vi "4_5.vi"() -> ()   [LabVIEW 2012]
panel:
  in  "stop":bool
  in  "OK Button":bool
  out "-":dbl[](array[numeric])
  out "+":dbl[](array[numeric])
  in  "Array":dbl[](array[numeric])
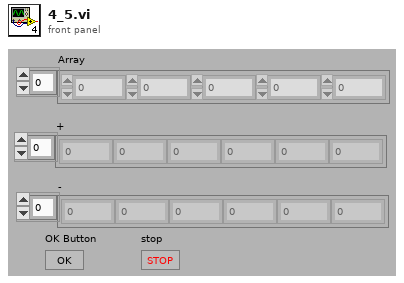
[diagram p1: front panel]
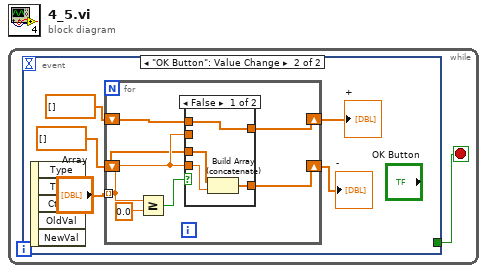
[diagram p0: block diagram]
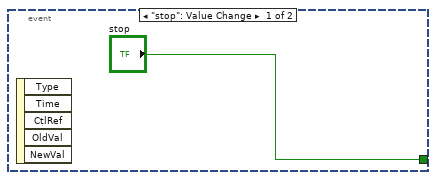
[diagram p2: hidden frame]
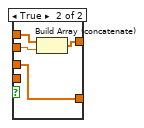
[diagram p3: hidden frame]
diagram:
  n1 = while {
    stop <- w1 stop-if-true
    n2 = event shown="[1] \"OK Button\": Value Change" {
      selector: _ -> [_ _]
      dyn-events: _ -> [_ _]
      timeout: _ -> [_ _]
      tunnel: ["stop" _] -> w1
      event "stop": Value Change {
        n3 = event-data() -> ()  [unwired: 1 in, 5 out]
      }
      event "OK Button": Value Change {
        n4 = event-data() -> ()  [unwired: 1 in, 5 out]
        n5 = for {
          tunnel: "Array" -> [w13] mode=indexing
          shift-right: [w10] -> w5
          shift-left: dbl[] [] -> [w11]
          shift-right: [w8] -> w7
          shift-left: dbl[] [] -> [w9]
          n6 = Greater Or Equal?(x=w13, y=0.0) -> (x >= y?=w14:bool)
          n7 = case shown="False" w14 {
            tunnel: w13 -> [_ w20]
            tunnel: w13 -> [w17 _]
            tunnel: w11 -> [w18 w22]
            tunnel: [w18 w21] -> w10
            tunnel: w9 -> [w16 w19]
            tunnel: [w15 w19] -> w8
            frame False {
              n8 = Build Array (concatenate)(w16, w17) -> (w15:dbl[])
            }
            frame True {
              n9 = Build Array (concatenate)(w22, w20) -> (w21:dbl[])
            }
          }
        }
        "+" <- w5
        "-" <- w7
      }
    }
  }
